vi "ConvertVoltToDegree.vi"(10 "Tension":dbl) -> (2 "Température":dbl)   [LabVIEW 2018]
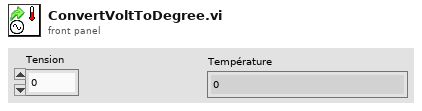
[diagram p1: front panel]
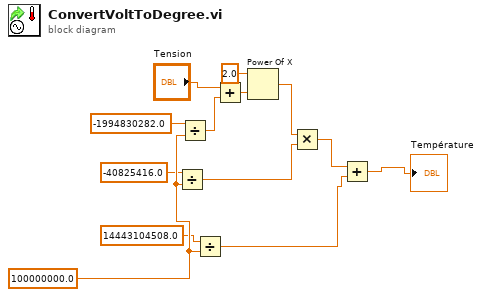
[diagram p0: block diagram]
diagram:
  w8 = 100000000.0
  n1 = Divide(x=-40825416.0, y=w8) -> (x/y=w12:dbl)
  n2 = Divide(x=-1994830282.0, y=w8) -> (x/y=w13:dbl)
  n3 = Divide(x=14443104508.0, y=w8) -> (x/y=w11:dbl)
  n4 = Add(x="Tension", y=w13) -> (x+y=w3:dbl)
  n5 = Power Of X(1:w3, 2:2.0 ("y")) -> (0:w2:dbl)
  n6 = Multiply(x=w2, y=w12) -> (x*y=w10:dbl)
  n7 = Add(x=w10, y=w11) -> (x+y=→"Température":dbl)
